vi "Accept.vi"(8 "error in (no error)":errorcluster, 10 "Accepted Runes":string, 11 "JSON Lexer in":refnum<class "JSON Lexer.lvclass">) -> (0 "error out":errorcluster, 1 "EOF":bool, 2 "Accepted?":bool, 3 "JSON Lexer out":refnum<class "JSON Lexer.lvclass">, 4 "Rune":string)   [LabVIEW 2019, in "JKI JSON Serialization.lvlib" / "JSON Lexer.lvclass"]
doc: "JKI JSON 1.1.10.37\nTomi Maila - JKI\nCopyright (c) 2017, JKI"
uses:
  JSON Lexer.lvclass
  JSON Lexer.lvclass/JSON Lexer.ctl
  Unicode/UTF-8 String/UTF-8 String.lvclass/UTF-8 String.ctl
  Unicode/UTF-8 String/Index Rune as UTF-8 Substring.vi
  Unicode/UTF-8 String/Next Rune As UTF-8 Substring.vi
  Unicode/UTF-8 String/Bytes In Rune.vi
  <vilib>/Utility/error.llb/Error Cluster From Error Code.vi
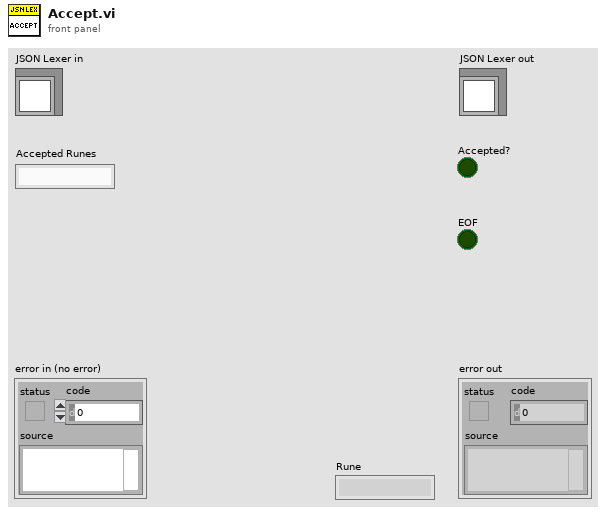
[diagram p1: front panel]
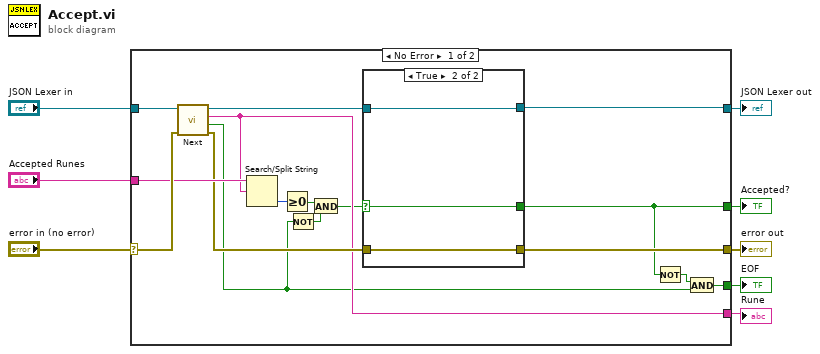
[diagram p0: block diagram]
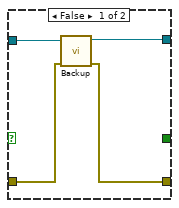
[diagram p2: hidden frame]
diagram:
  n1 = case shown="No Error" "error in (no error)" {
    selector: "error in (no error)" -> [w23 w33]
    tunnel: [w19 w33] -> w7
    tunnel: [w17 w32] -> w5
    tunnel: "JSON Lexer in" -> [w24 w32]
    tunnel: "Accepted Runes" -> [w22 _]
    tunnel: [w13 _] -> w3
    tunnel: [w15 _] -> w2
    tunnel: [w16 _] -> w1
    frame No Error {
      n2 = call "Next.vi"("error in (no error)"=w23, "JSON Lexer in"=w24) -> ("error out"=w20:errorcluster, "EOF"=w10:bool, "Rune"=w16:string, "JSON Lexer out"=w18:refnum<class "JSON Lexer.lvclass">)  [unwired: 6 in]
      n3 = Search/Split String(string=w22, search string/char (-)=w16) -> (offset of match=w21:i32)  [unwired: 1 in, 2 out]
      n4 = Greater Or Equal To 0?(x=w21) -> (x >= 0?=w12:bool)
      n5 = Not(x=w10) -> (.not. x?=w11:bool)
      n6 = And(x=w12, y=w11) -> (x .and. y?=w9:bool)
      n7 = case shown="True" w9 {
        selector: w9 -> [_ w29]
        tunnel: w20 -> [w27 w31]
        tunnel: [w26 w31] -> w19
        tunnel: w18 -> [w28 w30]
        tunnel: [w25 w30] -> w17
        tunnel: [_ w29] -> w13
        frame False {
          n8 = call "Backup.vi"("error in (no error)"=w27, "JSON Lexer in"=w28) -> ("error out"=w26:errorcluster, "JSON Lexer out"=w25:refnum<class "JSON Lexer.lvclass">)  [unwired: 8 in]
        }
        frame True {
        }
      }
      n9 = Not(x=w13) -> (.not. x?=w14:bool)
      n10 = And(x=w14, y=w10) -> (x .and. y?=w15:bool)
    }
    frame Error {
    }
  }
  "error out" <- w7
  "JSON Lexer out" <- w5
  "Accepted?" <- w3
  "EOF" <- w2
  "Rune" <- w1
